vi "Test Coffee Shop Add Barista.vi"(8 "error in (no error)":errorcluster, 11 "Coffee Shop Test In":refnum<class "Coffee Shop Test.lvclass">) -> (0 "error out":errorcluster, 3 "Coffee Shop Test Out":refnum<class "Coffee Shop Test.lvclass">)   [LabVIEW 2020, in "Coffee Shop Test.lvclass"]
uses:
  Coffee Shop Test.lvclass
  C:/Program Files (x86)/National Instruments/LabVIEW 2020/vi.lib/Astemes/LUnit/Test Case.lvclass
  Processes/Coffee Shop/Coffee Shop.lvclass
  C:/Program Files (x86)/National Instruments/LabVIEW 2020/vi.lib/Astemes/Triarc Framework/Process/Process.lvclass
  C:/Program Files (x86)/National Instruments/LabVIEW 2020/vi.lib/Astemes/Triarc Framework/Application/Application.lvclass
  <vilib>/Astemes/Triarc Framework/Process/Process.lvclass/Process.ctl
  <vilib>/Astemes/Triarc Framework/Application/Application.lvclass/Application.ctl
  <vilib>/Astemes/LUnit/Test Case.lvclass/Test Case.ctl
  97ddfd79-0019-43cf-87e6-eb0eb55d66ea.vi
  <vilib>/Astemes/Triarc Framework/Process/Public/Lifecycle/Get Lifecycle State.vi
  <vilib>/Astemes/Triarc Framework/Application/Private/Retrieve Process from App.vi
  <vilib>/Astemes/Triarc Framework/Application/Private/Parse Process Name.vi
  <vilib>/Astemes/Triarc Framework/Application/Private/Get Process from Map.vi
  <vilib>/Astemes/Triarc Framework/Process/Private/SubVIs/Wait for finish.vi
  <vilib>/Astemes/Triarc Framework/Process/Private/SubVIs/Set Lifecycle State.vi
  <vilib>/Astemes/Triarc Framework/Process/Protected/Messaging/Send Message.vi
  <vilib>/Astemes/LUnit/Palette/Pass.vi
  <vilib>/Astemes/LUnit/Palette/Fail.vi
  <vilib>/Astemes/LUnit/Compare Variants.vi
  <vilib>/Astemes/LUnit/Describe Comparison.vi
  <vilib>/Astemes/LUnit/Set Assertion Type.vi
  <vilib>/Utility/error.llb/Clear Errors.vi
  <vilib>/Astemes/Triarc Framework/Process/Protected/Messaging/Request Message.vi
  <vilib>/Astemes/Triarc Framework/Application/Private/Add Process to Map.vi
  <vilib>/AdvancedString/Delimited String to 1D String Array.vi
  <vilib>/Astemes/Triarc Framework/Process/Private/SubVIs/Handle Debug Data.vi
  <vilib>/Astemes/LUnit/Add test result.vi
  <vilib>/Astemes/LUnit/Variant to string.vi
  <vilib>/Astemes/Triarc Framework/Process/Private/SubVIs/Enqueue Request Message.vi
  <vilib>/Astemes/Triarc Framework/Logging/Log Debug.vi
  <vilib>/AdvancedString/1D String Array to Delimited String.vi
  <vilib>/Utility/High Resolution Relative Seconds.vi
  <vilib>/Astemes/LUnit/LUnit Record Assertion Result.vi
  <vilib>/Astemes/LUnit/LUnit Aggregate Assertion Results.vi
  <vilib>/Astemes/LUnit/Method Result/LUnit Merge Status.vi
  <vilib>/Astemes/LUnit/LUnit Concatenate result strings.vi
  <vilib>/Astemes/Triarc Framework/Application/Application.lvclass
  <vilib>/Utility/error.llb/Error Cluster From Error Code.vi
  <vilib>/Astemes/Triarc Framework/Process/Private/SubVIs/Wait for Response Message.vi
  <vilib>/Utility/Data Type/Get Type Information.vi
  <vilib>/Utility/LVClass/Get LV Class Name.vi
  <vilib>/Astemes/Triarc Framework/Process/Process.lvclass
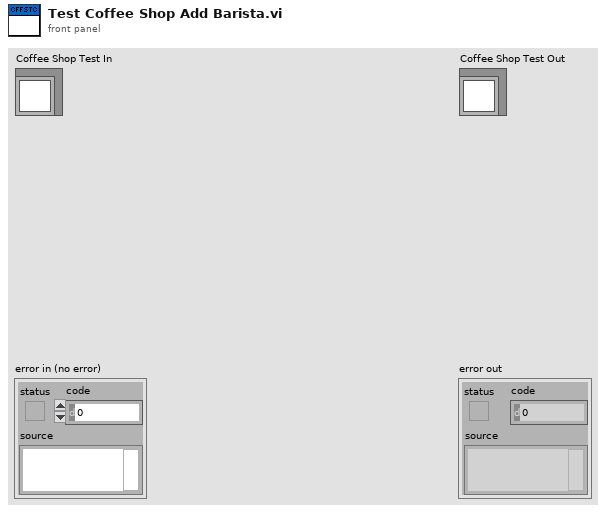
[diagram p1: front panel]
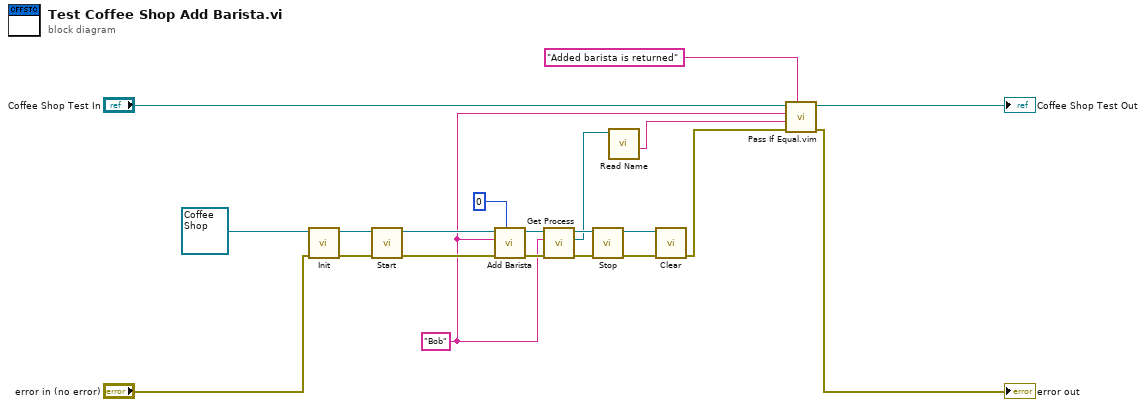
[diagram p0: block diagram]
diagram:
  w4 = "Bob" ("Name")
  n1 = call-dynamic "Init.vi"("error in (no error)"="error in (no error)", "Process In"=refnum<class "Coffee Shop.lvclass"> refnum ("Coffee Shop.lvclass")) -> ("error out"=w19:errorcluster, "Process Out"=w20:refnum<class "Coffee Shop.lvclass">)  [unwired: 8 in]
  n2 = call <vilib>:"Start.vi"("error in (no error)"=w19, "Process In"=w20) -> ("error out"=w14:errorcluster, "Process Out"=w13:refnum<class "Coffee Shop.lvclass">)  [unwired: 7 in, 1 out]
  n3 = call "Add Barista.vi"("Time Scale [ms]"=u32 0, "error in (no error)"=w14, "Name"=w4, "Coffee Shop in"=w13) -> ("error out"=w15:errorcluster, "Coffee Shop out"=w6:refnum<class "Coffee Shop.lvclass">)  [unwired: 6 in]
  n4 = call <vilib>:"Get Process.vi"("error in (no error)"=w15, "Process Name"=w4, "Application In"=w6) -> ("error out"=w7:errorcluster, "App Process"=w3:refnum<class "Process.lvclass">, "Application Out"=w5:refnum<class "Coffee Shop.lvclass">)  [unwired: 6 in]
  n5 = call <vilib>:"Stop.vi"("error in (no error)"=w7, "Process In"=w5) -> ("error out"=w17:errorcluster, "Process Out"=w18:refnum<class "Coffee Shop.lvclass">)  [unwired: 7 in, 1 out]
  n6 = call <vilib>:"Read Name.vi"("Process In"=w3) -> ("Name"=w2:string)  [unwired: 7 in, 3 out]
  n7 = call-dynamic "Clear.vi"("error in (no error)"=w17, "Application In"=w18) -> ("error out"=w10:errorcluster)  [unwired: 9 in]
  n8 = call "Pass If Equal.vim"("Description"="Added barista is returned", "error in (no error)"=w10, "Actual"=w2, "Expected"=w4, "LUnit Test Case In"="Coffee Shop Test In") -> ("error out"=→"error out":errorcluster, "LUnit Test Case Out"=→"Coffee Shop Test Out":refnum<class "Coffee Shop Test.lvclass">)  [unwired: 5 in]
